vi "Test Generate Mock Class Creates lvclass File.vi"(8 "error in (no error)":errorcluster, 11 "Test Case In":refnum<class "Mock Class Generator Test.lvclass">) -> (0 "error out":errorcluster, 3 "Test Case Out":refnum<class "Mock Class Generator Test.lvclass">)   [LabVIEW 2020, in "Mock Class Generator Test.lvclass"]
uses:
  Mock Class Generator Test.lvclass
  C:/Program Files (x86)/National Instruments/LabVIEW 2020/vi.lib/Astemes/LUnit/Test Case.lvclass
  <vilib>/Astemes/LUnit/Test Case.lvclass/Test Case.ctl
  <vilib>/Astemes/LUnit/Append Pass Result.vi
  <vilib>/Astemes/LUnit/Append Fail Result.vi
  source/Mock Class Generator/Mock Class Generator.lvclass
  <vilib>/Astemes/LUnit/Test Case.lvclass
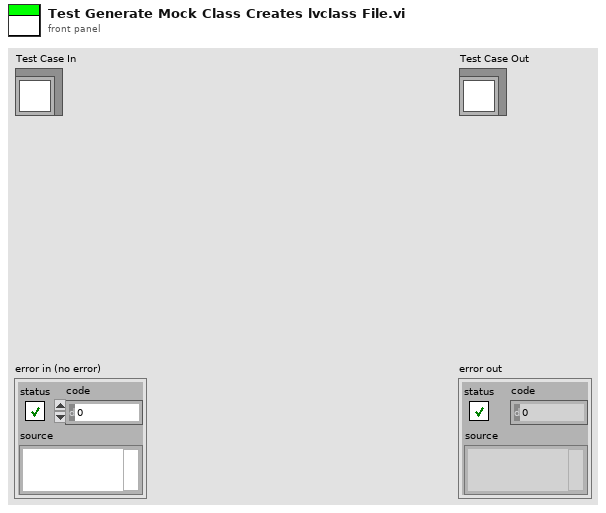
[diagram p1: front panel]
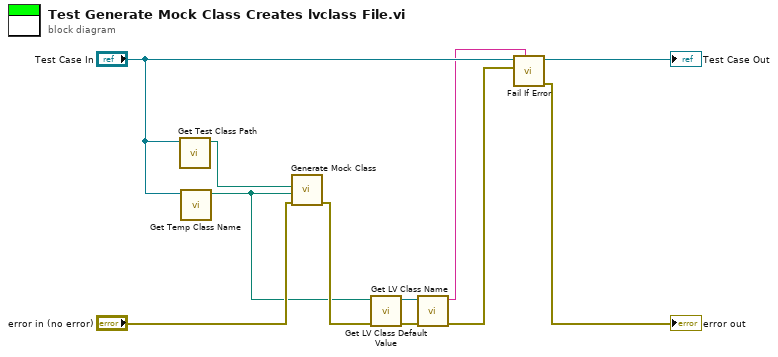
[diagram p0: block diagram]
diagram:
  n1 = call "Get Test Class Path.vi"("Mock Class Generator Test in"="Test Case In") -> ("Test Class Path"=w9:path)  [unwired: 10 in]
  n2 = call "Get Temp Class Name.vi"("Mock Class Generator Test in"="Test Case In") -> ("Test Class Path"=w4:path)  [unwired: 10 in]
  n3 = call "Generate Mock Class.vi"("error in (no error)"="error in (no error)", "Destination Class Path"=w4, "Source Class Path"=w9) -> ("error out"=w6:errorcluster)  [unwired: 8 in]
  n4 = call <vilib>:"Get LV Class Default Value.vi"("error in (no error)"=w6, "class path"=w4) -> ("error out"=w5:errorcluster, "object"=w3:refnum<class>)  [unwired: 8 in]
  n5 = call <vilib>:"Get LV Class Name.vi"("error in (no error)"=w5, "object"=w3) -> ("error out"=w1:errorcluster, "class name"=w2:string)  [unwired: 8 in]
  n6 = call <vilib>:"Fail If Error.vi"("Description"=w2, "Assert error"=w1, "LUnit Test Case In"="Test Case In") -> ("error out"=→"error out":errorcluster, "LUnit Test Case Out"=→"Test Case Out":refnum<class "Mock Class Generator Test.lvclass">)  [unwired: 7 in]
